vi "FSR_Query.vi"(0 "System no.":i32=1 min=1 max=4 step=1, 2 "Axes to query":string[](array[string]), 3 "Query all axes?":bool, 5 "error in":errorcluster) -> (14 "FSF successful?":bool[](array[boolean]), 19 "error out":errorcluster)   [LabVIEW 2020]
doc: "Indicates whether the find surface procedure for queried axes was successful.\n\nC-413:"
panel:
  # "Returns the result of the find surface procedure (FSF)."
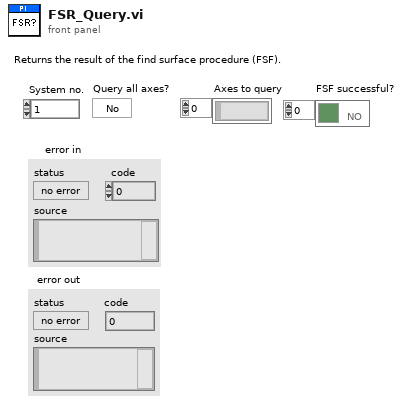
[diagram p1: front panel]
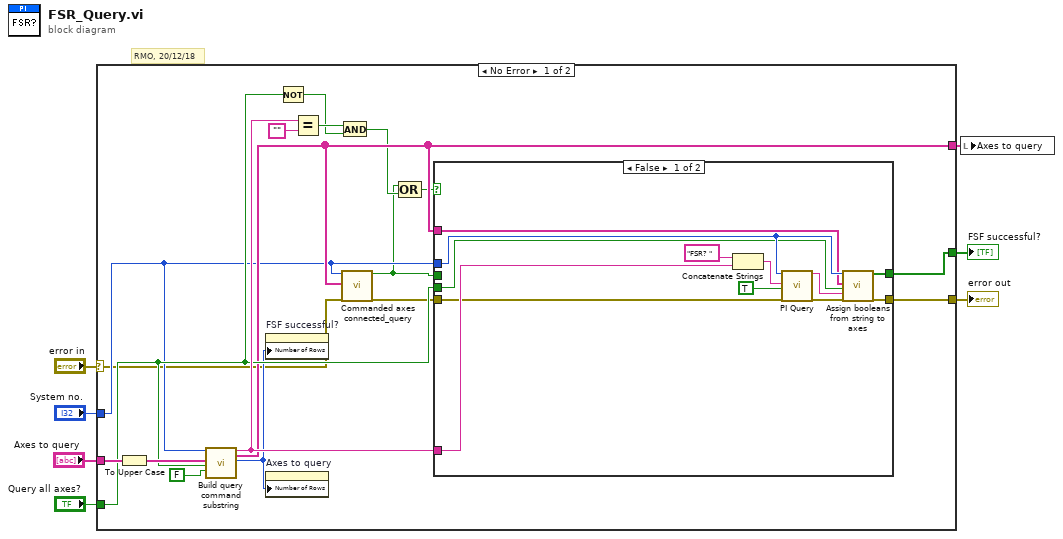
[diagram p0: block diagram]
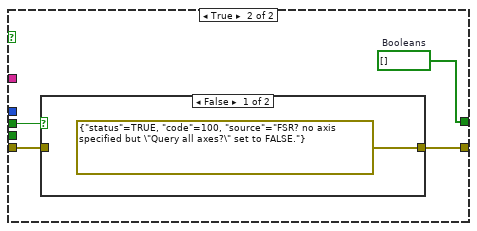
[diagram p2: hidden frame]
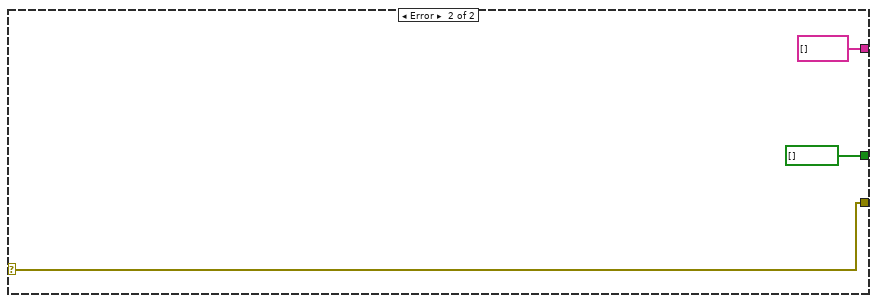
[diagram p4: hidden frame]
diagram:
  # "RMO, 20/12/18"
  n1 = case shown="No Error" "error in" {
    selector: "error in" -> [w8 w44]
    tunnel: [w25 bool[] [] ("Booleans")] -> w7
    tunnel: "Axes to query" -> [w24 _]
    tunnel: [w15 w44] -> w5
    tunnel: "System no." -> [w12 _]
    tunnel: [w13 string[] [] ("Axes to query out")] -> w3
    tunnel: "Query all axes?" -> [w20 _]
    frame No Error {
      n2 = To Upper Case(1:w24) -> (0:w22:string[])
      n3 = call "Build query command substring.vi"("System no."=w12, "Axes to query in"=w22, "Query\nAll axes?"=w20, "For all axes: use\nAxis identifier?"=FALSE ("For all axes: use\nAxis identifier?")) -> ("Command substring"=w21:string, "Axes to query out"=w13:string[], "Number of rows"=w17:u32)  [unwired: 2 in, 11 out]
      n4 = property on="FSF successful?" class="Arr (strict)"("Number of Rows"=w17) -> ()  [unwired: 2 in, 2 out]
      n5 = property on="Axes to query" class="Arr (strict)"("Number of Rows"=w17) -> ()  [unwired: 2 in, 2 out]
      n6 = Not(x=w20) -> (.not. x?=w18:bool)
      n7 = Equal?(x=w21, y="" ("x")) -> (x = y?=w19:bool)
      n8 = And(x=w19, y=w18) -> (x .and. y?=w10:bool)
      n9 = call "Commanded axes connected_query.vi"("System no."=w12, "Commanded axes"=w13, "error in"=w8) -> ("Controller error"=w9:bool, "error out"=w14:errorcluster)  [unwired: 1 in, 14 out]
      n10 = Compound Arithmetic op=OR(w9, w10) -> (w11:bool)
      n11 = case shown="False" w11 {
        tunnel: [w34 w40] -> w25
        tunnel: w14 -> [w28 w39]
        tunnel: w21 -> [w33 _]
        tunnel: w12 -> [w32 _]
        tunnel: w13 -> [w31 _]
        tunnel: w20 -> [w30 _]
        tunnel: [w29 w41] -> w15
        tunnel: w9 -> [_ w38]
        frame False {
          n12 = Concatenate Strings("FSR? ", w33) -> (w35:string)
          n13 = call "PI Query.vi"("System no."=w32, "String to send"=w35, "Attach termination char.?"=TRUE ("Attach Linefeed?"), "error in"=w28) -> ("String read"=w26:string, "error out"=w27:errorcluster)  [unwired: 3 in, 11 out]
          n14 = call "Assign booleans from string to axes.vi"("System no."=w32, "Queried axes"=w31, "All axes queried?"=w30, "Input String"=w26, "error in"=w27) -> ("Booleans"=w34:bool[], "error out"=w29:errorcluster)  [unwired: 13 out]
        }
        frame True {
          w40 = bool[] []  # Booleans
          n15 = case shown="False" w38 {
            tunnel: [errorcluster {"status"=TRUE, "code"=100, "source"="FSR? no axis specified but \"Query all axes?\" set to FALSE."} ("error out") w43] -> w41
            tunnel: w39 -> [_ w43]
            frame False {
            }
            frame True {
            }
          }
        }
      }
    }
    frame Error {
    }
  }
  "error out" <- w5
  "FSF successful?" <- w7
  n16 = local write "Axes to query"(w3) -> ()
